vi "Begin.vi"(8 "error in":errorcluster) -> (0 "error out":errorcluster)   [LabVIEW 2020]
doc: "Called before other user functions, this VI is expected to open initial I/O refnums, load in file data, and do all program initialization. Notice that the <B>error out</B> terminal is simply used for data flow. Wiring it to other structures or subVIs ensures that this VI runs first."
uses:
  <vilib>/Rock Robotics/WPI/DriverStation/WPI_DriverStationRobotMode2.ctl
  <vilib>/Rock Robotics/WPI/Joystick/WPI_JoystickDeviceEnum.ctl
  <vilib>/Rock Robotics/WPI/ThirdParty/Phoenix-LabVIEW/Motor Controller/Controls/CTRE_Phoenix_MotorControl_NeutralMode.ctl
  <vilib>/Rock Robotics/WPI/SafetyOutput/WPI_SafetyOutputConfigMenu.ctl
  <vilib>/Rock Robotics/SystemInterfaces/DIO/FPGA_DIOChannel.ctl
  Robot Global Data.vi
  <vilib>/Rock Robotics/Network Tables/NT Write String Array.vi
  <vilib>/Rock Robotics/WPI/RobotDrive/WPI_RobotDriveOpen4MotorWithExistingMotors.vi
  <vilib>/Rock Robotics/Network Tables/NT Write Number.vi
  GlobalVariables.vi
  <vilib>/Rock Robotics/WPI/Counter/WPI_CounterDigitalInputToDigitalSource.vi
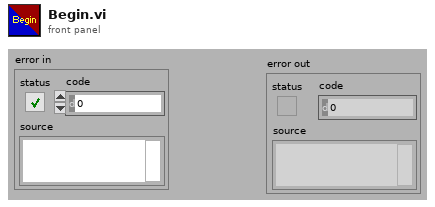
[diagram p1: front panel]
types:
  T1 = typedef "FPGA_DIOChannel.ctl" = enum8{"DIO 0", "DIO 1", "DIO 2", "DIO 3", "DIO 4", "DIO 5", "DIO 6", "DIO 7", "DIO 8", "DIO 9", "DIO MXP 0", "DIO MXP 1", "DIO MXP 2", "DIO MXP 3", "DIO MXP 4", "DIO MXP 5", "DIO MXP 6", "DIO MXP 7", "DIO MXP 8", "DIO MXP 9", "DIO MXP 10", "DIO MXP 11", "DIO MXP 12", "DIO MXP 13", "DIO MXP 14", "DIO MXP 15", "SPI Port CS1", "SPI Port CS2", "SPI Port CS3", "SPI Port MISO", "SPI Port MOSI", "Invalid"}
  T2 = typedef "CTRE_Phoenix_MotorControl_NeutralMode.ctl" = enum8{"EEPROMSetting", "Override to Coast", "Override to Brake"}
  T3 = typedef "WPI_SafetyOutputConfigMenu.ctl" = enum16{"Enable", "Disable"}
  T4 = typedef "WPI_JoystickDeviceEnum.ctl" = enum16{"USB 0", "USB 1", "USB 2", "USB 3", "USB 4", "USB 5"}
  T5 = typedef "WPI_DriverStationRobotMode2.ctl" = enum16{"Autonomous Disabled", "Autonomous Enabled", "Teleop Disabled", "Teleop Enabled", "Disconnected", "Finish", "Test Disabled", "Test Enabled", "Emergency Stopped"}
  T6 = typedef "WPI_DigitalInputDevRef.ctl" = cluster{"DevStatus":errorcluster, "DIO Channel":T1}
  T7 = typedef "FPGA_CounterEncoderSourceConvertionLVSourceType.ctl" = cluster{"DevStatus":errorcluster, "AnalogTriggerMode?":bool, "DigitalMode":cluster{"DIO Channel":T8}, "AnalogTriggerMode":cluster{"AnalogTriggerIndex":T9, "OutputType":T10}}
  T8 = typedef "FPGA_DIODigitalSourceChannel.ctl" = enum8{"DIO 0", "DIO 1", "DIO 2", "DIO 3", "DIO 4", "DIO 5", "DIO 6", "DIO 7", "DIO 8", "DIO 9", "DIO MXP 0", "DIO MXP 1", "DIO MXP 2", "DIO MXP 3", "DIO MXP 4", "DIO MXP 5", "DIO MXP 6", "DIO MXP 7", "DIO MXP 8", "DIO MXP 9", "DIO MXP 10", "DIO MXP 11", "DIO MXP 12", "DIO MXP 13", "DIO MXP 14", "DIO MXP 15", "SPI Port CS1", "SPI Port CS2", "SPI Port CS3", "SPI Port MISO", "SPI Port MOSI", "Disabled"}
  T9 = typedef "FPGA_AnalogTriggerIndex.ctl" = enum8{"Trig 0", "Trig 1", "Trig 2", "Trig 3", "Trig 4", "Trig 5", "Trig 6", "Trig 7", "Invalid"}
  T10 = typedef "FPGA_AnalogTriggerOutType.ctl" = enum16{"InWindow", "TriggerState", "Rising", "Falling"}
  T11 = typedef "WPI_MotorControlDeviceRef.ctl" = cluster{"DeviceStatus":errorcluster, "Type":T12, "PWM":cluster{"PWM Channel":T13, "DeadBand":T14}, "CAN":cluster{"Device Number":u8, "SetOutput VI Ref":variant, "GetOutput VI Ref":variant, "Enable VI Ref":variant, "Disable VI Ref":variant, "Data":variant}, "Invert":bool, "DIO PWM":cluster{"PWM \"Enable\" Channel":T13, "DIOChannel":T1, "PWM Rate":dbl}}
  T12 = typedef "WPI_MotorControlType.ctl" = enum16{"PWM", "CAN", "DIO PWM"}
  T13 = typedef "FPGA_DIOPWMChannel.ctl" = enum8{"PWM 0", "PWM 1", "PWM 2", "PWM 3", "PWM 4", "PWM 5", "PWM 6", "PWM 7", "PWM 8", "PWM 9", "PWM MXP 0", "PWM MXP 1", "PWM MXP 2", "PWM MXP 3", "PWM MXP 4", "PWM MXP 5", "PWM MXP 6", "PWM MXP 7", "PWM MXP 8", "PWM MXP 9", "Invalid"}
  T14 = typedef "WPI_PWMDeadband.ctl" = cluster{"Name":string, "maxPositivePwm":i32, "minPositivePwm":i32, "centerPwm":i32, "maxNegativePwm":i32, "minNegativePwm":i32, "angularRange":u16}
  T15 = typedef "WPI_EncoderDevRef.ctl" = cluster{"DevStatus":errorcluster, "EncoderIndex":T16, "CounterIndex":T17, "DistancePerCount":dbl, "Decoding Type":T18}
  T16 = typedef "FPGA_EncoderIdx.ctl" = enum8{"Enc 0", "Enc 1", "Enc 2", "Enc 3", "Enc 4", "Enc 5", "Enc 6", "Enc 7", "Invalid"}
  T17 = typedef "FPGA_CounterCtrSystemIndex.ctl" = enum8{"Ctr 0", "Ctr 1", "Ctr 2", "Ctr 3", "Ctr 4", "Ctr 5", "Ctr 6", "Ctr 7", "Invalid"}
  T18 = typedef "WPI_EncoderType.ctl" = enum16{"1x", "2x", "4x"}
  T19 = typedef "WPI_RobotDriveDevRef.ctl" = cluster{"DevStatus":errorcluster, "Motors[]":T11[], "Square Inputs":bool, "Max Output":dbl}
  T20 = typedef "WPI_JoystickDevRef.ctl" = cluster{"Device":T4}
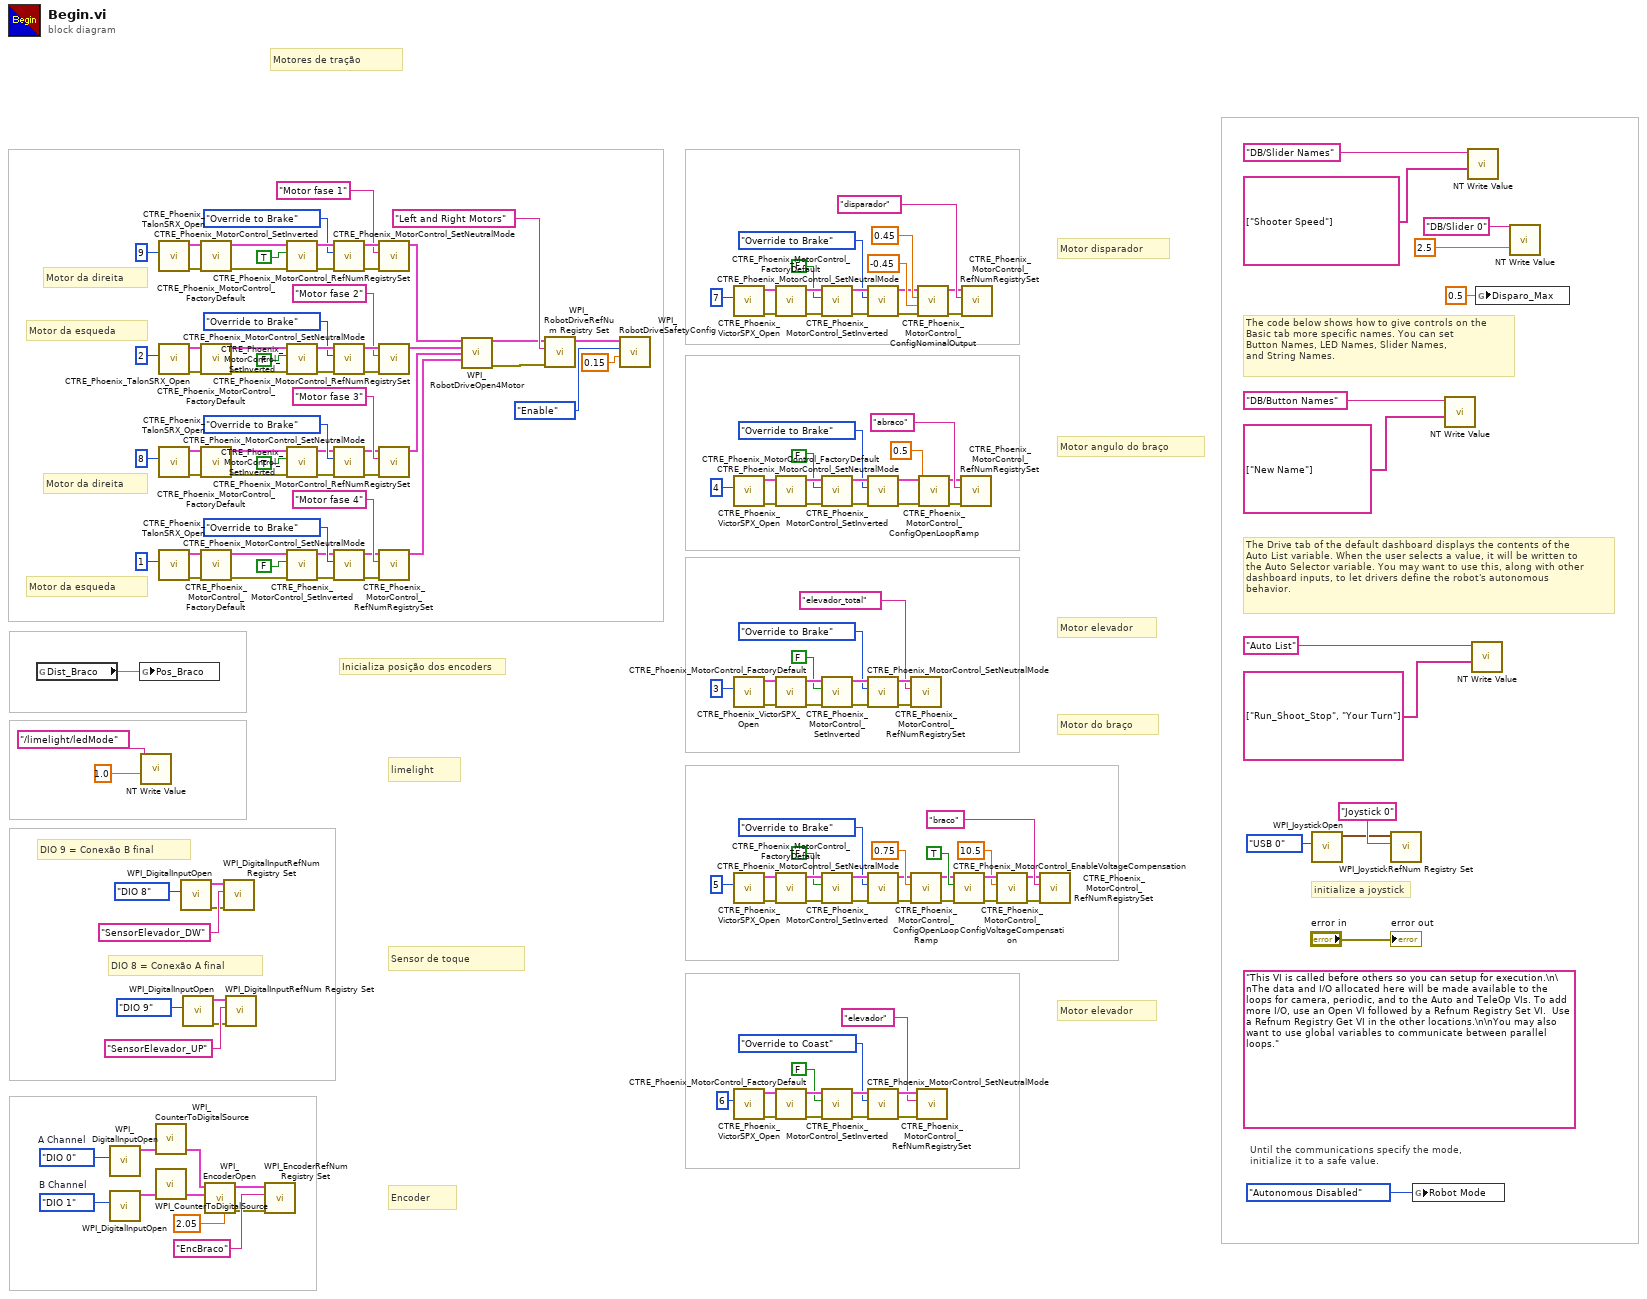
[diagram p0: block diagram]
diagram:
  w8 = FPGA_DIOChannel."DIO 1"  # B Channel
  w7 = FPGA_DIOChannel."DIO 0"  # A Channel
  (unwired) "This VI is called before others so you can setup for execution.\n\nThe data and I/O allocated here will be made available to the loops for camera, periodic, and to the Auto and TeleOp VIs. To add more I/O, use an Open VI followed by a Refnum Registry Set VI.  Use a Refnum Registry Get VI in the other locations.\n\nYou may also want to use global variables to communicate between parallel loops."
  # "Encoder"
  # "Inicializa posição dos encoders"
  # "Sensor de toque"
  # "limelight"
  # "Motores de tração"
  # "DIO 8 = Conexão A final"
  # "DIO 9 = Conexão B final"
  # "Motor elevador"
  # "Motor do braço"
  # "Motor angulo do braço"
  # "Motor elevador"
  # "Motor disparador"
  # "Motor da esqueda"
  # "Motor da direita"
  # "Motor da esqueda"
  # "Motor da direita"
  # "The Drive tab of the default dashboard displays the contents of the\nAuto List variable. When the user selects a value, it will be written to\nthe Auto Selector variable. You may want to use this, along with other\ndashboard inputs, to let drivers define the robot's autonomous\nbehavior."
  # "The code below shows how to give controls on the\nBasic tab more specific names. You can set\nButton Names, LED Names, Slider Names,\nand String Names."
  # "initialize a joystick"
  # "Until the communications specify the mode,\ninitialize it to a safe value."
  n1 = global read "GlobalVariables.vi" "Dist_Braco"() -> (w16:dbl)
  n2 = call <vilib>:"WPI_DigitalInputOpen.vi"("DIO Channel"=w7) -> ("DigitalInputDevRef"=w5:T6)  [unwired: 1 in, 9 out]
  n3 = call <vilib>:"WPI_DigitalInputOpen.vi"("DIO Channel"=w8) -> ("DigitalInputDevRef"=w6:T6)  [unwired: 1 in, 9 out]
  n4 = global write "GlobalVariables.vi" "Pos_Braco"(w16) -> ()
  n5 = call-poly <vilib>:"NT Write Value.vi"("Numeric"=1.0, "Name"="/limelight/ledMode") -> ()  [unwired: 9 in, 1 out]
  n6 = call-poly <vilib>:"WPI_CounterToDigitalSource.vi"("DigitalInputDevRef"=w5) -> ("Digital Source"=w9:T7)  [unwired: 6 out]
  n7 = call-poly <vilib>:"WPI_CounterToDigitalSource.vi"("DigitalInputDevRef"=w6) -> ("Digital Source"=w10:T7)  [unwired: 6 out]
  n8 = call <vilib>:"CTRE_Phoenix_TalonSRX_Open.vi"("Device Number"=u8 9) -> ("error out"=w123:errorcluster, "PhoenixMotorControlDevRef"=w122:T11)  [unwired: 9 in]
  n9 = call <vilib>:"CTRE_Phoenix_TalonSRX_Open.vi"("Device Number"=u8 2) -> ("error out"=w159:errorcluster, "PhoenixMotorControlDevRef"=w158:T11)  [unwired: 9 in]
  n10 = call <vilib>:"CTRE_Phoenix_TalonSRX_Open.vi"("Device Number"=u8 8) -> ("error out"=w126:errorcluster, "PhoenixMotorControlDevRef"=w127:T11)  [unwired: 9 in]
  n11 = call <vilib>:"CTRE_Phoenix_TalonSRX_Open.vi"("Device Number"=u8 1) -> ("error out"=w138:errorcluster, "PhoenixMotorControlDevRef"=w139:T11)  [unwired: 9 in]
  n12 = call <vilib>:"WPI_DigitalInputOpen.vi"("DIO Channel"=FPGA_DIOChannel."DIO 8") -> ("error out"=w21:errorcluster, "DigitalInputDevRef"=w23:T6)  [unwired: 9 in]
  n13 = call <vilib>:"WPI_DigitalInputOpen.vi"("DIO Channel"=FPGA_DIOChannel."DIO 9") -> ("error out"=w17:errorcluster, "DigitalInputDevRef"=w19:T6)  [unwired: 9 in]
  n14 = call <vilib>:"CTRE_Phoenix_MotorControl_FactoryDefault.vi"("error in"=w123, "PhoenixMotorControlDevRef"=w122) -> ("error out"=w120:errorcluster, "PhoenixMotorControlDevRef"=w121:T11)  [unwired: 8 in]
  n15 = call <vilib>:"CTRE_Phoenix_MotorControl_FactoryDefault.vi"("error in"=w159, "PhoenixMotorControlDevRef"=w158) -> ("error out"=w156:errorcluster, "PhoenixMotorControlDevRef"=w157:T11)  [unwired: 8 in]
  n16 = call <vilib>:"CTRE_Phoenix_MotorControl_FactoryDefault.vi"("error in"=w126, "PhoenixMotorControlDevRef"=w127) -> ("error out"=w129:errorcluster, "PhoenixMotorControlDevRef"=w128:T11)  [unwired: 8 in]
  n17 = call <vilib>:"CTRE_Phoenix_MotorControl_FactoryDefault.vi"("error in"=w138, "PhoenixMotorControlDevRef"=w139) -> ("error out"=w141:errorcluster, "PhoenixMotorControlDevRef"=w140:T11)  [unwired: 8 in]
  n18 = call <vilib>:"WPI_EncoderOpen.vi"("DistancePerCount"=2.05, "BSource"=w10, "ASource"=w9) -> ("error out"=w2:errorcluster, "EncoderDevRef"=w4:T15)  [unwired: 7 in]
  n19 = call <vilib>:"WPI_DigitalInputRefNum Registry Set.vi"("error in (no error)"=w21, "refnum name"="SensorElevador_DW", "DigitalInputDevRef"=w23) -> ()  [unwired: 7 in, 2 out]
  n20 = call <vilib>:"WPI_DigitalInputRefNum Registry Set.vi"("error in (no error)"=w17, "refnum name"="SensorElevador_UP", "DigitalInputDevRef"=w19) -> ()  [unwired: 7 in, 2 out]
  n21 = call <vilib>:"WPI_EncoderRefNum Registry Set.vi"("error in (no error)"=w2, "refnum name"="EncBraco", "EncoderDevRef"=w4) -> ()  [unwired: 7 in, 2 out]
  n22 = call <vilib>:"CTRE_Phoenix_MotorControl_SetInverted.vi"("error in (no error)"=w120, "Invert?"=TRUE, "PhoenixMotorControlDevRef"=w121) -> ("error out"=w117:errorcluster, "PhoenixMotorControlDevRef"=w118:T11)  [unwired: 7 in]
  n23 = call <vilib>:"CTRE_Phoenix_MotorControl_SetInverted.vi"("error in (no error)"=w156, "Invert?"=FALSE, "PhoenixMotorControlDevRef"=w157) -> ("error out"=w153:errorcluster, "PhoenixMotorControlDevRef"=w154:T11)  [unwired: 7 in]
  n24 = call <vilib>:"CTRE_Phoenix_MotorControl_SetInverted.vi"("error in (no error)"=w129, "Invert?"=TRUE, "PhoenixMotorControlDevRef"=w128) -> ("error out"=w132:errorcluster, "PhoenixMotorControlDevRef"=w131:T11)  [unwired: 7 in]
  n25 = call <vilib>:"CTRE_Phoenix_MotorControl_SetInverted.vi"("error in (no error)"=w141, "Invert?"=FALSE, "PhoenixMotorControlDevRef"=w140) -> ("error out"=w144:errorcluster, "PhoenixMotorControlDevRef"=w143:T11)  [unwired: 7 in]
  n26 = call <vilib>:"CTRE_Phoenix_MotorControl_SetNeutralMode.vi"("error in (no error)"=w117, "Motor Control Neutral Mode"=CTRE_Phoenix_MotorControl_NeutralMode."Override to Brake", "PhoenixMotorControlDevRef"=w118) -> ("error out"=w113:errorcluster, "PhoenixMotorControlDevRef"=w115:T11)  [unwired: 7 in]
  n27 = call <vilib>:"CTRE_Phoenix_MotorControl_SetNeutralMode.vi"("error in (no error)"=w153, "Motor Control Neutral Mode"=CTRE_Phoenix_MotorControl_NeutralMode."Override to Brake", "PhoenixMotorControlDevRef"=w154) -> ("error out"=w149:errorcluster, "PhoenixMotorControlDevRef"=w151:T11)  [unwired: 7 in]
  n28 = call <vilib>:"CTRE_Phoenix_MotorControl_SetNeutralMode.vi"("error in (no error)"=w132, "Motor Control Neutral Mode"=CTRE_Phoenix_MotorControl_NeutralMode."Override to Brake", "PhoenixMotorControlDevRef"=w131) -> ("error out"=w136:errorcluster, "PhoenixMotorControlDevRef"=w134:T11)  [unwired: 7 in]
  n29 = call <vilib>:"CTRE_Phoenix_MotorControl_SetNeutralMode.vi"("error in (no error)"=w144, "Motor Control Neutral Mode"=CTRE_Phoenix_MotorControl_NeutralMode."Override to Brake", "PhoenixMotorControlDevRef"=w143) -> ("error out"=w148:errorcluster, "PhoenixMotorControlDevRef"=w146:T11)  [unwired: 7 in]
  n30 = call <vilib>:"CTRE_Phoenix_MotorControl_RefNumRegistrySet.vi"("error in (no error)"=w113, "refnum name"="Motor fase 1", "PhoenixMotorControlDevRef"=w115) -> ("PhoenixMotorControlDevRef"=w112:T11)  [unwired: 7 in, 1 out]
  n31 = call <vilib>:"CTRE_Phoenix_MotorControl_RefNumRegistrySet.vi"("error in (no error)"=w149, "refnum name"="Motor fase 2", "PhoenixMotorControlDevRef"=w151) -> ("PhoenixMotorControlDevRef"=w110:T11)  [unwired: 7 in, 1 out]
  n32 = call <vilib>:"CTRE_Phoenix_MotorControl_RefNumRegistrySet.vi"("error in (no error)"=w136, "refnum name"="Motor fase 3", "PhoenixMotorControlDevRef"=w134) -> ("PhoenixMotorControlDevRef"=w111:T11)  [unwired: 7 in, 1 out]
  n33 = call <vilib>:"CTRE_Phoenix_MotorControl_RefNumRegistrySet.vi"("error in (no error)"=w148, "refnum name"="Motor fase 4", "PhoenixMotorControlDevRef"=w146) -> ("PhoenixMotorControlDevRef"=w109:T11)  [unwired: 7 in, 1 out]
  n34 = call-poly <vilib>:"WPI_RobotDriveOpen4Motor.vi"("Rear Left Motor Dev Ref"=w112, "Rear Right Motor Dev Ref"=w110, "Front Left Motor Dev Ref"=w111, "Front Right Motor Dev Ref"=w109) -> ("RobotDriveDevRef"=w105:T19, "error out"=w104:errorcluster)  [unwired: 10 in]
  n35 = call <vilib>:"WPI_RobotDriveRefNum Registry Set.vi"("error in (no error)"=w104, "refnum name"="Left and Right Motors", "RobotDriveDevRef"=w105) -> ("RobotDriveDevRef"=w108:T19)  [unwired: 7 in, 1 out]
  n36 = call <vilib>:"WPI_RobotDriveSafetyConfig.vi"("timeout (s)"=0.15, "mode"=WPI_SafetyOutputConfigMenu."Enable", "RobotDriveDevRef"=w108) -> ()  [unwired: 7 in, 2 out]
  n37 = call <vilib>:"CTRE_Phoenix_VictorSPX_Open.vi"("Device Number"=u8 7) -> ("error out"=w99:errorcluster, "PhoenixMotorControlDevRef"=w100:T11)  [unwired: 9 in]
  n38 = call <vilib>:"CTRE_Phoenix_VictorSPX_Open.vi"("Device Number"=u8 4) -> ("error out"=w77:errorcluster, "PhoenixMotorControlDevRef"=w78:T11)  [unwired: 9 in]
  n39 = call <vilib>:"CTRE_Phoenix_VictorSPX_Open.vi"("Device Number"=u8 3) -> ("error out"=w57:errorcluster, "PhoenixMotorControlDevRef"=w58:T11)  [unwired: 9 in]
  n40 = call <vilib>:"CTRE_Phoenix_VictorSPX_Open.vi"("Device Number"=u8 5) -> ("error out"=w67:errorcluster, "PhoenixMotorControlDevRef"=w68:T11)  [unwired: 9 in]
  n41 = call <vilib>:"CTRE_Phoenix_VictorSPX_Open.vi"("Device Number"=u8 6) -> ("error out"=w89:errorcluster, "PhoenixMotorControlDevRef"=w90:T11)  [unwired: 9 in]
  n42 = call <vilib>:"CTRE_Phoenix_MotorControl_FactoryDefault.vi"("error in"=w99, "PhoenixMotorControlDevRef"=w100) -> ("error out"=w97:errorcluster, "PhoenixMotorControlDevRef"=w98:T11)  [unwired: 8 in]
  n43 = call <vilib>:"CTRE_Phoenix_MotorControl_FactoryDefault.vi"("error in"=w77, "PhoenixMotorControlDevRef"=w78) -> ("error out"=w75:errorcluster, "PhoenixMotorControlDevRef"=w76:T11)  [unwired: 8 in]
  n44 = call <vilib>:"CTRE_Phoenix_MotorControl_FactoryDefault.vi"("error in"=w57, "PhoenixMotorControlDevRef"=w58) -> ("error out"=w55:errorcluster, "PhoenixMotorControlDevRef"=w56:T11)  [unwired: 8 in]
  n45 = call <vilib>:"CTRE_Phoenix_MotorControl_FactoryDefault.vi"("error in"=w67, "PhoenixMotorControlDevRef"=w68) -> ("error out"=w65:errorcluster, "PhoenixMotorControlDevRef"=w66:T11)  [unwired: 8 in]
  n46 = call <vilib>:"CTRE_Phoenix_MotorControl_FactoryDefault.vi"("error in"=w89, "PhoenixMotorControlDevRef"=w90) -> ("error out"=w87:errorcluster, "PhoenixMotorControlDevRef"=w88:T11)  [unwired: 8 in]
  n47 = call <vilib>:"CTRE_Phoenix_MotorControl_SetInverted.vi"("error in (no error)"=w97, "Invert?"=FALSE, "PhoenixMotorControlDevRef"=w98) -> ("error out"=w94:errorcluster, "PhoenixMotorControlDevRef"=w95:T11)  [unwired: 7 in]
  n48 = call <vilib>:"CTRE_Phoenix_MotorControl_SetInverted.vi"("error in (no error)"=w75, "Invert?"=FALSE, "PhoenixMotorControlDevRef"=w76) -> ("error out"=w72:errorcluster, "PhoenixMotorControlDevRef"=w73:T11)  [unwired: 7 in]
  n49 = call <vilib>:"CTRE_Phoenix_MotorControl_SetInverted.vi"("error in (no error)"=w55, "Invert?"=FALSE, "PhoenixMotorControlDevRef"=w56) -> ("error out"=w50:errorcluster, "PhoenixMotorControlDevRef"=w53:T11)  [unwired: 7 in]
  n50 = call <vilib>:"CTRE_Phoenix_MotorControl_SetInverted.vi"("error in (no error)"=w65, "Invert?"=FALSE, "PhoenixMotorControlDevRef"=w66) -> ("error out"=w62:errorcluster, "PhoenixMotorControlDevRef"=w63:T11)  [unwired: 7 in]
  n51 = call <vilib>:"CTRE_Phoenix_MotorControl_SetInverted.vi"("error in (no error)"=w87, "Invert?"=FALSE, "PhoenixMotorControlDevRef"=w88) -> ("error out"=w82:errorcluster, "PhoenixMotorControlDevRef"=w85:T11)  [unwired: 7 in]
  n52 = call <vilib>:"CTRE_Phoenix_MotorControl_SetNeutralMode.vi"("error in (no error)"=w94, "Motor Control Neutral Mode"=CTRE_Phoenix_MotorControl_NeutralMode."Override to Brake", "PhoenixMotorControlDevRef"=w95) -> ("error out"=w34:errorcluster, "PhoenixMotorControlDevRef"=w35:T11)  [unwired: 7 in]
  n53 = call <vilib>:"CTRE_Phoenix_MotorControl_SetNeutralMode.vi"("error in (no error)"=w72, "Motor Control Neutral Mode"=CTRE_Phoenix_MotorControl_NeutralMode."Override to Brake", "PhoenixMotorControlDevRef"=w73) -> ("error out"=w27:errorcluster, "PhoenixMotorControlDevRef"=w28:T11)  [unwired: 7 in]
  n54 = call <vilib>:"CTRE_Phoenix_MotorControl_SetNeutralMode.vi"("error in (no error)"=w50, "Motor Control Neutral Mode"=CTRE_Phoenix_MotorControl_NeutralMode."Override to Brake", "PhoenixMotorControlDevRef"=w53) -> ("error out"=w51:errorcluster, "PhoenixMotorControlDevRef"=w52:T11)  [unwired: 7 in]
  n55 = call <vilib>:"CTRE_Phoenix_MotorControl_SetNeutralMode.vi"("error in (no error)"=w62, "Motor Control Neutral Mode"=CTRE_Phoenix_MotorControl_NeutralMode."Override to Brake", "PhoenixMotorControlDevRef"=w63) -> ("error out"=w32:errorcluster, "PhoenixMotorControlDevRef"=w33:T11)  [unwired: 7 in]
  n56 = call <vilib>:"CTRE_Phoenix_MotorControl_SetNeutralMode.vi"("error in (no error)"=w82, "Motor Control Neutral Mode"=CTRE_Phoenix_MotorControl_NeutralMode."Override to Coast", "PhoenixMotorControlDevRef"=w85) -> ("error out"=w83:errorcluster, "PhoenixMotorControlDevRef"=w84:T11)  [unwired: 7 in]
  n57 = call <vilib>:"CTRE_Phoenix_MotorControl_RefNumRegistrySet.vi"("error in (no error)"=w51, "refnum name"="elevador_total", "PhoenixMotorControlDevRef"=w52) -> ()  [unwired: 7 in, 2 out]
  n58 = call <vilib>:"CTRE_Phoenix_MotorControl_ConfigOpenLoopRamp.vi"("error in (no error)"=w32, "secondsFromNeutralToFull"=0.75, "PhoenixMotorControlDevRef"=w33) -> ("error out"=w39:errorcluster, "PhoenixMotorControlDevRef"=w40:T11)  [unwired: 7 in]
  n59 = call <vilib>:"CTRE_Phoenix_MotorControl_RefNumRegistrySet.vi"("error in (no error)"=w83, "refnum name"="elevador", "PhoenixMotorControlDevRef"=w84) -> ()  [unwired: 7 in, 2 out]
  n60 = call <vilib>:"CTRE_Phoenix_MotorControl_ConfigNominalOutput.vi"("error in (no error)"=w34, "Reverse Nominal Percent Output"=-0.45, "Forward Nominal Percent Output"=0.45, "PhoenixMotorControlDevRef"=w35) -> ("error out"=w45:errorcluster, "PhoenixMotorControlDevRef"=w46:T11)  [unwired: 6 in]
  n61 = call <vilib>:"CTRE_Phoenix_MotorControl_ConfigOpenLoopRamp.vi"("error in (no error)"=w27, "secondsFromNeutralToFull"=0.5, "PhoenixMotorControlDevRef"=w28) -> ("error out"=w25:errorcluster, "PhoenixMotorControlDevRef"=w26:T11)  [unwired: 7 in]
  n62 = call <vilib>:"CTRE_Phoenix_MotorControl_EnableVoltageCompensation.vi"("error in (no error)"=w39, "Enable Voltage Compensation?"=TRUE, "PhoenixMotorControlDevRef"=w40) -> ("error out"=w43:errorcluster, "PhoenixMotorControlDevRef"=w44:T11)  [unwired: 7 in]
  n63 = call <vilib>:"CTRE_Phoenix_MotorControl_RefNumRegistrySet.vi"("error in (no error)"=w25, "refnum name"="abraco", "PhoenixMotorControlDevRef"=w26) -> ()  [unwired: 7 in, 2 out]
  n64 = call <vilib>:"CTRE_Phoenix_MotorControl_RefNumRegistrySet.vi"("error in (no error)"=w45, "refnum name"="disparador", "PhoenixMotorControlDevRef"=w46) -> ()  [unwired: 7 in, 2 out]
  n65 = call <vilib>:"CTRE_Phoenix_MotorControl_ConfigVoltageCompensation.vi"("error in (no error)"=w43, "Saturation Voltage"=10.5, "PhoenixMotorControlDevRef"=w44) -> ("error out"=w30:errorcluster, "PhoenixMotorControlDevRef"=w31:T11)  [unwired: 7 in]
  n66 = call <vilib>:"CTRE_Phoenix_MotorControl_RefNumRegistrySet.vi"("error in (no error)"=w30, "refnum name"="braco", "PhoenixMotorControlDevRef"=w31) -> ()  [unwired: 7 in, 2 out]
  n67 = call <vilib>:"WPI_JoystickOpen.vi"("JoystickDevice"=WPI_JoystickDeviceEnum."USB 0") -> ("JoystickDevRef"=w167:T20)  [unwired: 10 in]
  n68 = call <vilib>:"WPI_JoystickRefNum Registry Set.vi"("refnum name"="Joystick 0", "JoystickDevRef"=w167) -> ()  [unwired: 8 in, 2 out]
  n69 = global write "Robot Global Data.vi" "Robot Mode"(WPI_DriverStationRobotMode2."Autonomous Disabled" ("Robot Mode")) -> ()
  n70 = call-poly <vilib>:"NT Write Value.vi"("String Array"=string[] ["New Name"], "Name"="DB/Button Names") -> ()  [unwired: 9 in, 1 out]
  n71 = call-poly <vilib>:"NT Write Value.vi"("String Array"=string[] ["Shooter Speed"], "Name"="DB/Slider Names") -> ()  [unwired: 9 in, 1 out]
  n72 = call-poly <vilib>:"NT Write Value.vi"("String Array"=string[] ["Run_Shoot_Stop", "Your Turn"], "Name"="Auto List") -> ()  [unwired: 9 in, 1 out]
  n73 = global write "GlobalVariables.vi" "Disparo_Max"(0.5 ("Disparo_Max")) -> ()
  n74 = call-poly <vilib>:"NT Write Value.vi"("Numeric"=2.5, "Name"="DB/Slider 0") -> ()  [unwired: 9 in, 1 out]
  "error out" <- "error in"
